vi "Initiate Stream.vi"(0 "niUsrpRio Session":T1={"Global Settings Register Bus"=refnum, "Radio 0 Settings Register Bus"=refnum, "Rx NI-USRP session"="", "Tx NI-USRP session"="", "FPGA Interface"=refnum, "RIO Interface Number"=0, "EEPROM Header"={"Checksum"=0, "Product Code"=0, "Hardware Current Version"=0, "Hardware Oldest Compatible Version"=0, "EEPROM Map Current Version"=0, "EEPROM Map Oldest Compatible Version"=0, "User Password"="", "Pointer to Factory Header"=0, "Pointer to User Header"=0, "Recommended Interval"=0, "Number of Reserved Bytes"=9, "Number of Daughterboards"=0, "Daughterboard IDs"=[], "Daughterboard Serial Numbers"=[]}, "Device Data Header"={"Checksum"=0, "Number of Channels"=0, "Number of Gain Settings"=[], "Pointer to Characterization Data"=[], "Number of Reserved Bytes"=27, "Number of Frequencies"=[]}, "EEPROM Characterization Header"={"Checksum"=0, "Date"=timestamp(0 s since 1904-01-01), "Temperature"=0.0, "Misc. Info"="", "Pointer to Device Data Header"=0, "Number of Reserved Bytes"=28}, "Characterization Data"=[], "Characterization Data Valid?"=FALSE, "Radio 1 Settings Register Bus"=refnum, "Radio Settings Bus Semaphore"=refnum} {"Characterization Data"."Frequencies [Hz]" format="%#_6p"; "EEPROM Characterization Header"."Pointer to Device Data Header" format="%x"; "EEPROM Characterization Header"."Checksum" format="%x"; "Device Data Header"."Pointer to Characterization Data" format="%x"; "Device Data Header"."Checksum" format="%x"; "EEPROM Header"."Pointer to User Header" format="%x"; "EEPROM Header"."Pointer to Factory Header" format="%x"; "EEPROM Header"."Product Code" format="%x"; "EEPROM Header"."Checksum" format="%x"}, 1 "scope":string(combo)="rx", 11 "error in":errorcluster) -> (4 "niUsrpRio Session (out)":T1={"Global Settings Register Bus"=refnum, "Radio 0 Settings Register Bus"=refnum, "Rx NI-USRP session"="", "Tx NI-USRP session"="", "FPGA Interface"=refnum, "RIO Interface Number"=0, "EEPROM Header"={"Checksum"=0, "Product Code"=0, "Hardware Current Version"=0, "Hardware Oldest Compatible Version"=0, "EEPROM Map Current Version"=0, "EEPROM Map Oldest Compatible Version"=0, "User Password"="", "Pointer to Factory Header"=0, "Pointer to User Header"=0, "Recommended Interval"=0, "Number of Reserved Bytes"=9, "Number of Daughterboards"=0, "Daughterboard IDs"=[], "Daughterboard Serial Numbers"=[]}, "Device Data Header"={"Checksum"=0, "Number of Channels"=0, "Number of Gain Settings"=[], "Pointer to Characterization Data"=[], "Number of Reserved Bytes"=27, "Number of Frequencies"=[]}, "EEPROM Characterization Header"={"Checksum"=0, "Date"=timestamp(0 s since 1904-01-01), "Temperature"=0.0, "Misc. Info"="", "Pointer to Device Data Header"=0, "Number of Reserved Bytes"=28}, "Characterization Data"=[], "Characterization Data Valid?"=FALSE, "Radio 1 Settings Register Bus"=refnum, "Radio Settings Bus Semaphore"=refnum} {"Characterization Data"."Frequencies [Hz]" format="%#_6p"; "EEPROM Characterization Header"."Pointer to Device Data Header" format="%x"; "EEPROM Characterization Header"."Checksum" format="%x"; "Device Data Header"."Pointer to Characterization Data" format="%x"; "Device Data Header"."Checksum" format="%x"; "EEPROM Header"."Pointer to User Header" format="%x"; "EEPROM Header"."Pointer to Factory Header" format="%x"; "EEPROM Header"."Product Code" format="%x"; "EEPROM Header"."Checksum" format="%x"}, 15 "error out":errorcluster)   [LabVIEW 2013]
doc: "Initiates the stream. This is required before you acquire/generate data with the Fetch Rx Data or Write Tx Data VIs. Initiation includes resetting the Rx/Tx streams and the DSP.\n\n<B>Input Parameters</B>\n\n<B>niUsrpRio Session</B> is the object created by the Open VI and used as the session handle for the USRP RIO design library.\n\n<B>scope</B> is the channel on which stream is to be initiated. The options are \"rx/RF 0\", \"rx/RF 1\", \"tx/RF 0\", and \"tx/RF 1\".\n\n<B>error in</B> describes error conditions that occur before this node runs. This input provides standard 'error in' functionality.\n\n<B>Output Parameters</B>\n\n<B>niUsrpRio Session (out)</B> is the niUsrpRio session used in all subsequent USRP RIO design library host VIs.\n\n<B>error out</B> contains error information. This output provides standard 'error out' functionality."
uses:
  <instrlib>/niUsrpRio/Config/v1/Host/Public/niUsrpRio Session.ctl
  <instrlib>/_niInstr/Register Bus/v0/Host/Public/Register Bus Session.ctl
  <instrlib>/_niInstr/Register Bus/v0/Host/Private/Session Data.ctl
  <instrlib>/niUsrpRio/Config/v1/Host/Public/EEPROM Header.ctl
  <instrlib>/niUsrpRio/Config/v1/Host/Public/EEPROM Device Data Header.ctl
  <instrlib>/niUsrpRio/Config/v1/Host/Public/EEPROM Characterization Header.ctl
  <instrlib>/niUsrpRio/Config/v1/Host/Public/Characterization Data.ctl
  <instrlib>/niUsrpRio/Config/v1/Host/Public/IQ Imbalance.ctl
  Tx FPGA VI Reference.ctl
  Rx FPGA VI Reference.ctl
  <vilib>/Utility/error.llb/Error Cluster From Error Code.vi
  <vilib>/rvi/interface/common/niFpgaWaitOnOcc.vi
  <vilib>/rvi/errors/niLvFpgaAdjustHostInterfaceError.vi
  <vilib>/ErrorRing/Error Ring.xnode
  <vilib>/rvi/interface/nirviReadWriteControl/nirviReadWriteControl.xnode
  <vilib>/rvi/interface/Simulation/niFpgaSimulationCallBeginRW.vi
  NiFpgaLv.dll
  <instrlib>/niUsrpRio/Config/v1/Host/niUsrpRio Config v1 Host.lvlib
  <instrlib>/_niInstr/Register Bus/v0/Host/niInstr Register Bus v0 Host.lvlib
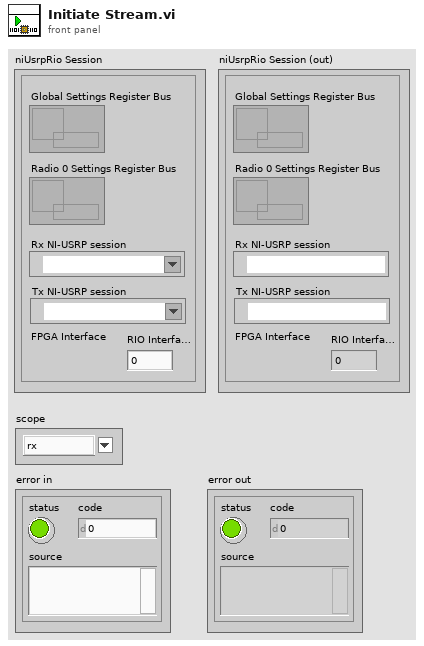
[diagram p1: front panel]
types:
  T1 = typedef "niUsrpRio Config v1 Host.lvlib/niUsrpRio Session.ctl" = cluster{"Global Settings Register Bus":T2, "Radio 0 Settings Register Bus":T2, "Rx NI-USRP session":refnum<k15>, "Tx NI-USRP session":refnum<k15>, "FPGA Interface":refnum<k20>, "RIO Interface Number":u32, "EEPROM Header":T3, "Device Data Header":T4, "EEPROM Characterization Header":T5, "Characterization Data":T6[], "Characterization Data Valid?":bool, "Radio 1 Settings Register Bus":T2, "Radio Settings Bus Semaphore":T8}
  T2 = typedef "niInstr Register Bus v0 Host.lvlib/Register Bus Session.ctl" = refnum<queue>
  T3 = typedef "niUsrpRio Config v1 Host.lvlib/EEPROM Header.ctl" = cluster{"Checksum":u32, "Product Code":u16, "Hardware Current Version":u16, "Hardware Oldest Compatible Version":u16, "EEPROM Map Current Version":u16, "EEPROM Map Oldest Compatible Version":u16, "User Password":string, "Pointer to Factory Header":u32, "Pointer to User Header":u32, "Recommended Interval":u16, "Number of Reserved Bytes":i32, "Number of Daughterboards":u8, "Daughterboard IDs":u16[], "Daughterboard Serial Numbers":string[]}
  T4 = typedef "niUsrpRio Config v1 Host.lvlib/EEPROM Device Data Header.ctl" = cluster{"Checksum":u32, "Number of Channels":u8, "Number of Gain Settings":u16[], "Pointer to Characterization Data":u32[], "Number of Reserved Bytes":i32, "Number of Frequencies":u16[]}
  T5 = typedef "niUsrpRio Config v1 Host.lvlib/EEPROM Characterization Header.ctl" = cluster{"Checksum":u32, "Date":timestamp, "Temperature":sgl, "Misc. Info":string, "Pointer to Device Data Header":u32, "Number of Reserved Bytes":i32}
  T6 = typedef "niUsrpRio Config v1 Host.lvlib/Characterization Data.ctl" = cluster{"Gains[dB]":dbl[], "Frequencies [Hz]":dbl[], "IQ Imbalance Table":T7[], "Measured Gains[dB]":dbl[][]}
  T7 = typedef "niUsrpRio Config v1 Host.lvlib/IQ Imbalance.ctl" = cluster{"Gain Imbalance [linear]":dbl, "Phase Imbalance [radians]":dbl, "Offset":cdb}
  T8 = typedef "Semaphore RefNum" = refnum<k1>
  T9 = typedef "niUsrpRio Config v1 Host.lvlib/Device Subfunction.ctl" = enum16{"rx", "tx"}
  T10 = typedef "niUsrpRio Config v1 Host.lvlib/RF Channel.ctl" = enum16{"0", "1", "All"}
  T11 = typedef "Tx FPGA VI Reference.ctl" = refnum<k20>
  T12 = typedef "Rx FPGA VI Reference.ctl" = refnum<k20>
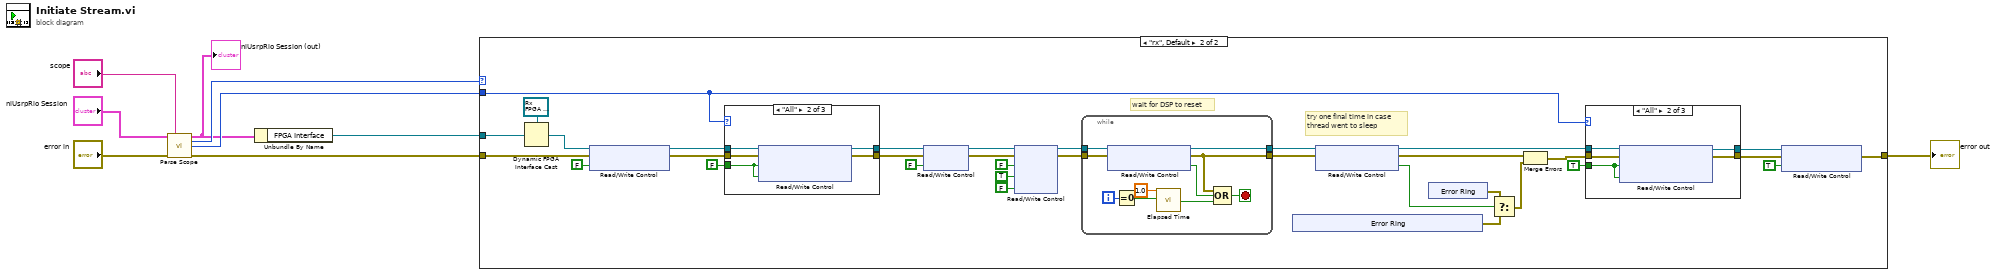
[diagram p0: block diagram]
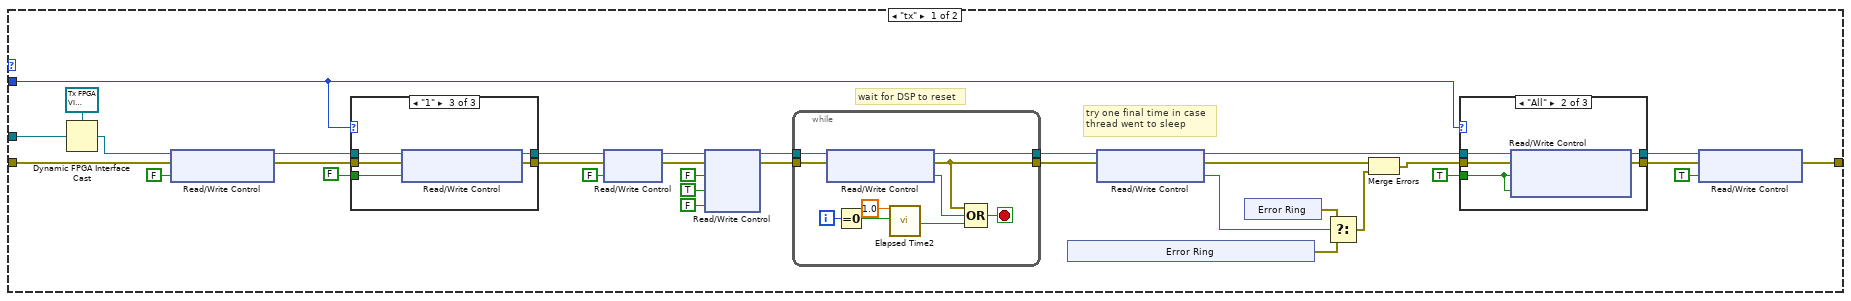
[diagram p2: hidden frame]
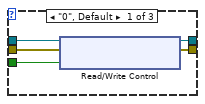
[diagram p3: hidden frame]
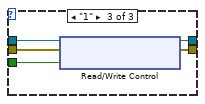
[diagram p4: hidden frame]
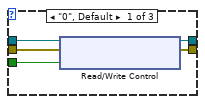
[diagram p5: hidden frame]
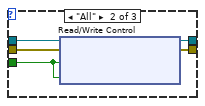
[diagram p6: hidden frame]
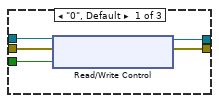
[diagram p7: hidden frame]
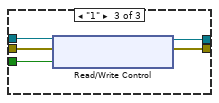
[diagram p8: hidden frame]
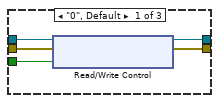
[diagram p9: hidden frame]
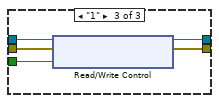
[diagram p10: hidden frame]
diagram:
  n1 = call <instrlib>:"Parse Scope.vi"("niUsrpRio Session"="niUsrpRio Session", "scope"="scope", "Error In"="error in") -> ("niUsrpRio Session (out)"=w1:T1, "Device Subfunction"=w7:T9, "Device Subfunction Channel"=w6:T10, "Error Out"=w4:errorcluster)  [unwired: 4 in, 5 out]
  "niUsrpRio Session (out)" <- w1
  n2 = Unbundle By Name(w1) -> ("FPGA Interface"=w5:refnum<k20>)
  n3 = case shown="\"rx\", Default" w7 {
    tunnel: w5 -> [w35 w121]
    tunnel: [w10 w89] -> w2
    tunnel: w4 -> [w18 w96]
    tunnel: w6 -> [w19 w101]
    frame "tx" {
      # "try one final time in case\nthread went to sleep"
      # "wait for DSP to reset"
      n4 = Dynamic FPGA Interface Cast(Session In=T11 refnum ("FPGA VI Reference Out"), Type=w35) -> (Session Out=w16:T11)
      n5 = xnode "Read/Write Control"("FPGA VI Reference In"=w16, "error in"=w18, "tx.enable trigger"=FALSE) -> ("FPGA VI Reference Out"=w15:T11, "error out"=w17:errorcluster)
      n6 = case shown="\"1\"" w19 {
        tunnel: w17 -> [w62 w67 w72]
        tunnel: w15 -> [w61 w66 w68]
        tunnel: [w60 w65 w70] -> w25
        tunnel: [w59 w64 w71] -> w24
        tunnel: FALSE ("tx.stream enabled") -> [w58 w63 w69]
        frame "0", Default {
          n7 = xnode "Read/Write Control"("FPGA VI Reference In"=w61, "error in"=w62, "tx 0.stream enabled"=w58) -> ("FPGA VI Reference Out"=w59:T11, "error out"=w60:errorcluster)
        }
        frame "All" {
          n8 = xnode "Read/Write Control"("FPGA VI Reference In"=w66, "error in"=w67, "tx 0.stream enabled"=w63, "tx 1.stream enabled"=w63) -> ("FPGA VI Reference Out"=w64:T11, "error out"=w65:errorcluster)
        }
        frame "1" {
          n9 = xnode "Read/Write Control"("FPGA VI Reference In"=w68, "error in"=w72, "tx 1.stream enabled"=w69) -> ("FPGA VI Reference Out"=w71:T11, "error out"=w70:errorcluster)
        }
      }
      n10 = xnode "Read/Write Control"("FPGA VI Reference In"=w24, "error in"=w25, "tx.abort"=FALSE) -> ("FPGA VI Reference Out"=w36:T11, "error out"=w37:errorcluster)
      n11 = xnode "Read/Write Control"("FPGA VI Reference In"=w36, "error in"=w37, "tx.reset"=FALSE, "tx.reset"=TRUE, "tx.reset"=FALSE) -> ("FPGA VI Reference Out"=w27:T11, "error out"=w26:errorcluster)
      n12 = while {
        tunnel: w27 -> [w88]
        tunnel: w26 -> [w87]
        tunnel: [w80] -> w34
        tunnel: [w79] -> w33
        i -> [w85]
        stop <- w81 stop-if-true
        n13 = xnode "Read/Write Control"("FPGA VI Reference In"=w88, "error in"=w87) -> ("FPGA VI Reference Out"=w79:T11, "error out"=w80:errorcluster, "tx.dsp reset done"=w83:bool)
        n14 = Equal To 0?(x=w85) -> (x = 0?=w86:bool)
        n15 = call "Elapsed Time2"("Time Target (s)"=1.0, "Reset"=w86) -> ("Time has Elapsed"=w82:bool)  [unwired: 10 in, 7 out]
        n16 = Compound Arithmetic op=OR(w80, w83, w82) -> (w81:bool)
      }
      n17 = xnode "Error Ring"() -> ("error out"=w28:errorcluster)
      n18 = xnode "Read/Write Control"("FPGA VI Reference In"=w33, "error in"=w34) -> ("FPGA VI Reference Out"=w21:T11, "error out"=w31:errorcluster, "tx.dsp reset done"=w32:bool)
      n19 = xnode "Error Ring"() -> ("error out"=w29:errorcluster)
      n20 = Select(t=w29, s=w32, f=w28) -> (s? t:f=w30:errorcluster)
      n21 = Merge Errors(w31, w30) -> (w20:errorcluster)
      n22 = case shown="\"All\"" w19 {
        tunnel: w20 -> [w47 w52 w57]
        tunnel: w21 -> [w46 w51 w53]
        tunnel: [w45 w50 w55] -> w11
        tunnel: [w44 w49 w56] -> w12
        tunnel: TRUE ("tx.stream enabled") -> [w43 w48 w54]
        frame "0", Default {
          n23 = xnode "Read/Write Control"("FPGA VI Reference In"=w46, "error in"=w47, "tx 0.stream enabled"=w43) -> ("FPGA VI Reference Out"=w44:T11, "error out"=w45:errorcluster)
        }
        frame "All" {
          n24 = xnode "Read/Write Control"("FPGA VI Reference In"=w51, "error in"=w52, "tx 0.stream enabled"=w48, "tx 1.stream enabled"=w48) -> ("FPGA VI Reference Out"=w49:T11, "error out"=w50:errorcluster)
        }
        frame "1" {
          n25 = xnode "Read/Write Control"("FPGA VI Reference In"=w53, "error in"=w57, "tx 1.stream enabled"=w54) -> ("FPGA VI Reference Out"=w56:T11, "error out"=w55:errorcluster)
        }
      }
      n26 = xnode "Read/Write Control"("FPGA VI Reference In"=w12, "error in"=w11, "tx.enable trigger"=TRUE) -> ("error out"=w10:errorcluster)  [unwired: 1 out]
    }
    frame "rx", Default {
      # "try one final time in case\nthread went to sleep"
      # "wait for DSP to reset"
      n27 = Dynamic FPGA Interface Cast(Session In=T12 refnum ("Type"), Type=w121) -> (Session Out=w97:T12)
      n28 = xnode "Read/Write Control"("FPGA VI Reference In"=w97, "error in"=w96, "rx.enable trigger"=FALSE) -> ("FPGA VI Reference Out"=w94:T12, "error out"=w95:errorcluster)
      n29 = case shown="\"All\"" w101 {
        tunnel: w94 -> [w141 w146 w151]
        tunnel: w95 -> [w140 w145 w150]
        tunnel: [w139 w144 w149] -> w107
        tunnel: [w138 w143 w148] -> w106
        tunnel: FALSE ("rx.stream enabled") -> [w137 w142 w147]
        frame "0", Default {
          n30 = xnode "Read/Write Control"("FPGA VI Reference In"=w141, "error in"=w140, "rx 0.stream enabled"=w137) -> ("FPGA VI Reference Out"=w139:T12, "error out"=w138:errorcluster)
        }
        frame "All" {
          n31 = xnode "Read/Write Control"("FPGA VI Reference In"=w146, "error in"=w145, "rx 0.stream enabled"=w142, "rx 1.stream enabled"=w142) -> ("FPGA VI Reference Out"=w144:T12, "error out"=w143:errorcluster)
        }
        frame "1" {
          n32 = xnode "Read/Write Control"("FPGA VI Reference In"=w151, "error in"=w150, "rx 1.stream enabled"=w147) -> ("FPGA VI Reference Out"=w149:T12, "error out"=w148:errorcluster)
        }
      }
      n33 = xnode "Read/Write Control"("FPGA VI Reference In"=w107, "error in"=w106, "rx.abort"=FALSE) -> ("FPGA VI Reference Out"=w104:T12, "error out"=w103:errorcluster)
      n34 = xnode "Read/Write Control"("FPGA VI Reference In"=w104, "error in"=w103, "rx.reset"=FALSE ("Acquisition.Reset"), "rx.reset"=TRUE, "rx.reset"=FALSE) -> ("FPGA VI Reference Out"=w108:T12, "error out"=w109:errorcluster)
      n35 = while {
        tunnel: w108 -> [w167]
        tunnel: w109 -> [w166]
        tunnel: [w159] -> w118
        tunnel: [w158] -> w117
        i -> [w164]
        stop <- w160 stop-if-true
        n36 = xnode "Read/Write Control"("FPGA VI Reference In"=w167, "error in"=w166) -> ("FPGA VI Reference Out"=w158:T12, "error out"=w159:errorcluster, "rx.dsp reset done"=w162:bool)
        n37 = Equal To 0?(x=w164) -> (x = 0?=w165:bool)
        n38 = call "Elapsed Time"("Time Target (s)"=1.0, "Reset"=w165) -> ("Time has Elapsed"=w161:bool)  [unwired: 10 in, 7 out]
        n39 = Compound Arithmetic op=OR(w159, w162, w161) -> (w160:bool)
      }
      n40 = xnode "Error Ring"() -> ("error out"=w112:errorcluster)
      n41 = xnode "Read/Write Control"("FPGA VI Reference In"=w117, "error in"=w118) -> ("FPGA VI Reference Out"=w102:T12, "error out"=w115:errorcluster, "rx.dsp reset done"=w116:bool)
      n42 = xnode "Error Ring"() -> ("error out"=w113:errorcluster)
      n43 = Select(t=w113, s=w116, f=w112) -> (s? t:f=w114:errorcluster)
      n44 = Merge Errors(w115, w114) -> (w100:errorcluster)
      n45 = case shown="\"All\"" w101 {
        tunnel: [w126 w131 w136] -> w91
        tunnel: [w125 w130 w135] -> w90
        tunnel: w102 -> [w124 w129 w134]
        tunnel: w100 -> [w123 w128 w133]
        tunnel: TRUE ("rx.stream enabled") -> [w122 w127 w132]
        frame "0", Default {
          n46 = xnode "Read/Write Control"("FPGA VI Reference In"=w124, "error in"=w123, "rx 0.stream enabled"=w122) -> ("FPGA VI Reference Out"=w126:T12, "error out"=w125:errorcluster)
        }
        frame "All" {
          n47 = xnode "Read/Write Control"("FPGA VI Reference In"=w129, "error in"=w128, "rx 0.stream enabled"=w127, "rx 1.stream enabled"=w127) -> ("FPGA VI Reference Out"=w131:T12, "error out"=w130:errorcluster)
        }
        frame "1" {
          n48 = xnode "Read/Write Control"("FPGA VI Reference In"=w134, "error in"=w133, "rx 1.stream enabled"=w132) -> ("FPGA VI Reference Out"=w136:T12, "error out"=w135:errorcluster)
        }
      }
      n49 = xnode "Read/Write Control"("FPGA VI Reference In"=w91, "error in"=w90, "rx.enable trigger"=TRUE) -> ("error out"=w89:errorcluster)  [unwired: 1 out]
    }
  }
  "error out" <- w2
